vi "Get Axis Position.vi"(4 "error in (no error)":errorcluster, 6 "Axis In":i16, 7 "Controller Reference":refnum<k7>) -> (0 "error out":errorcluster, 1 "Position Out":sgl, 2 "Axis Out":i16, 3 "Controller Reference out":refnum<k7>)   [LabVIEW 2015]
doc: "Gets the input Axis current Position."
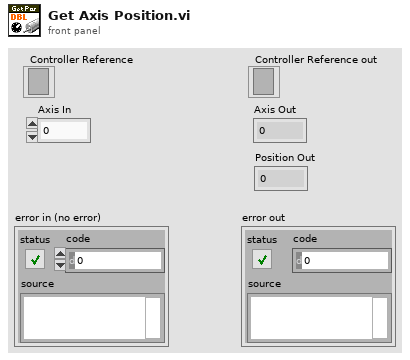
[diagram p1: front panel]
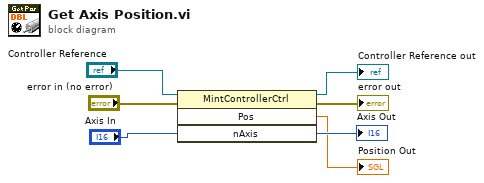
[diagram p0: block diagram]
diagram:
  n1 = invoke class="MintControllerCtrl" method="Pos"(reference="Controller Reference", error in="error in (no error)", "nAxis"="Axis In") -> (reference out=→"Controller Reference out":refnum<k7>, error out=→"error out":errorcluster, "Pos"=→"Position Out":sgl, "nAxis"=→"Axis Out":i16)  [unwired: 1 in]
